vi "Multi Dimensional Array Variant to Array of Variants.vi"(8 "error in (no error)":errorcluster, 11 "Array Variant":variant) -> (0 "error out":errorcluster, 3 "[Variant]":variant[](array[variant]))   [LabVIEW 2018, in "TwinCAT ADS.lvclass"]
uses:
  TwinCAT ADS.lvclass
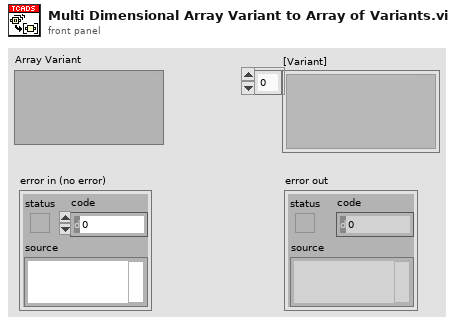
[diagram p1: front panel]
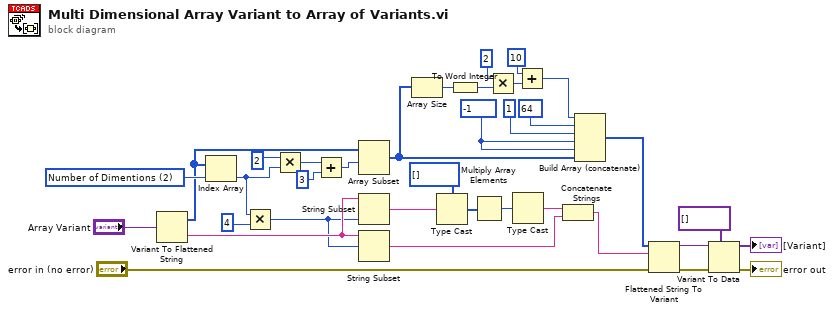
[diagram p0: block diagram]
diagram:
  w28 = i16 -1
  w35 = 2 items=["TD length", "Type Code", "Number of Dimentions"]
  n1 = Variant To Flattened String(Variant="Array Variant") -> (data string=w12:string, 1:w13:i16[])
  n2 = Index Array(array=w13, index=w35) -> (element=w1:i16)
  n3 = Multiply(x=w1, y=i16 4) -> (x*y=w9:i16)
  n4 = Multiply(x=i16 2 ("y"), y=w1) -> (x*y=w33:i16)
  n5 = Add(x=w33, y=i16 3) -> (x+y=w32:i16)
  n6 = Array Subset(array=w13, index=w32) -> (w16:i16[])  [unwired: 1 in]
  n7 = String Subset(string=w12, length (rest)=w9) -> (substring=w11:string)  [unwired: 1 in]
  n8 = String Subset(string=w12, offset (0)=w9) -> (substring=w5:string)  [unwired: 1 in]
  n9 = Array Size(array=w16) -> (size(s)=w17:i32)
  n10 = Type Cast(type=i32[] [] ("value"), x=w11) -> (*(type *) &x=w8:i32[])
  n11 = To Word Integer(number=w17) -> (16bit integer=w19:i16)
  n12 = Multiply Array Elements(1:w8) -> (0:w7:i32)
  n13 = Multiply(x=i16 2, y=w19) -> (x*y=w20:i16)
  n14 = Type Cast(x=w7) -> (*(type *) &x=w6:string)  [unwired: 1 in]
  n15 = Add(x=i16 10, y=w20) -> (x+y=w15:i16)
  n16 = Concatenate Strings(w6, w5) -> (w4:string)
  n17 = Build Array (concatenate)(w15, i16 64, i16 1 ("element"), w28, w28, w16) -> (w26:i16[])
  n18 = Flattened String To Variant(4:"error in (no error)", 6:w4, 7:w26) -> (0:w25:errorcluster, 3:w24:variant)
  n19 = Variant To Data(error in=w25, type=variant[] [], Variant=w24) -> (data=→"[Variant]":variant[], error out=→"error out":errorcluster)
